vi "Compare Ports.vi"(9 "refresh listbox":T8[](array[typedef]), 10 "new port":T1, 11 "old port":T1) -> (1 "refresh listbox out":T8[](array[typedef]))   [LabVIEW 2020, in "Ballard ARINC 429 System Explorer.lvlib" / "Implementation.lvlib"]
uses:
  Implementation.lvlib
  Types/Refresh Listbox.ctl
  Types/Refresh Symbols.ctl
  Shared/VS Channels Definition for All Labels on Hardware Channel.ctl
  Shared/VS Channels Definition for Label.ctl
  Shared/VS Channel Definition for Parameter.ctl
  Shared/Direction.ctl
  Shared/Parameter Definition.ctl
  Encoding and Decoding/Encoding.ctl
  Shared/Transfer Type.ctl
  Encoding and Decoding/Encoding and Decoding.lvlib
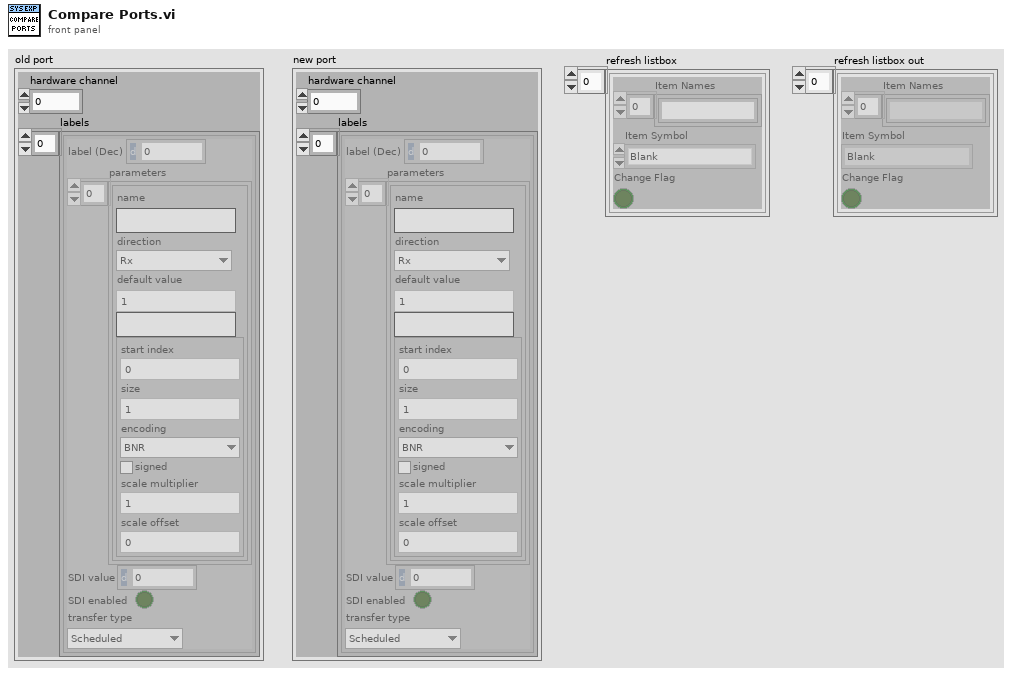
[diagram p1: front panel]
types:
  T1 = typedef "VS Channels Definition for All Labels on Hardware Channel.ctl" = cluster{"hardware channel":i32, "labels":T2[]}
  T2 = typedef "VS Channels Definition for Label.ctl" = cluster{"label (Dec)":u32, "parameters":T3[], "SDI value":u8, "SDI enabled":bool, "transfer type":T7}
  T3 = typedef "VS Channel Definition for Parameter.ctl" = cluster{"name":string, "direction":T4, "default value":dbl, "unit":string, "Parameter":T5}
  T4 = typedef "Direction.ctl" = enum16{"Rx", "Tx"}
  T5 = typedef "Parameter Definition.ctl" = cluster{"start index":i32, "size":i32, "encoding":T6, "signed":bool, "scale multiplier":dbl, "scale offset":dbl}
  T6 = typedef "Encoding and Decoding.lvlib/Encoding.ctl" = enum16{"BNR", "BCD", "Discrete"}
  T7 = typedef "Transfer Type.ctl" = enum16{"Scheduled", "Acyclic", "Block", "Strobe"}
  T8 = typedef "Ballard ARINC 429 System Explorer.lvlib/Implementation.lvlib/Refresh Listbox.ctl" = cluster{"Item Names":string[], "Item Symbol":T9, "Change Flag":bool}
  T9 = typedef "Ballard ARINC 429 System Explorer.lvlib/Implementation.lvlib/Refresh Symbols.ctl" = enum16{"Blank", "Port", "Incoming", "Outgoing", "Label", "Word", "Parameter", "ARINC-429", "Config Files", "Channel Spec", "Item"}
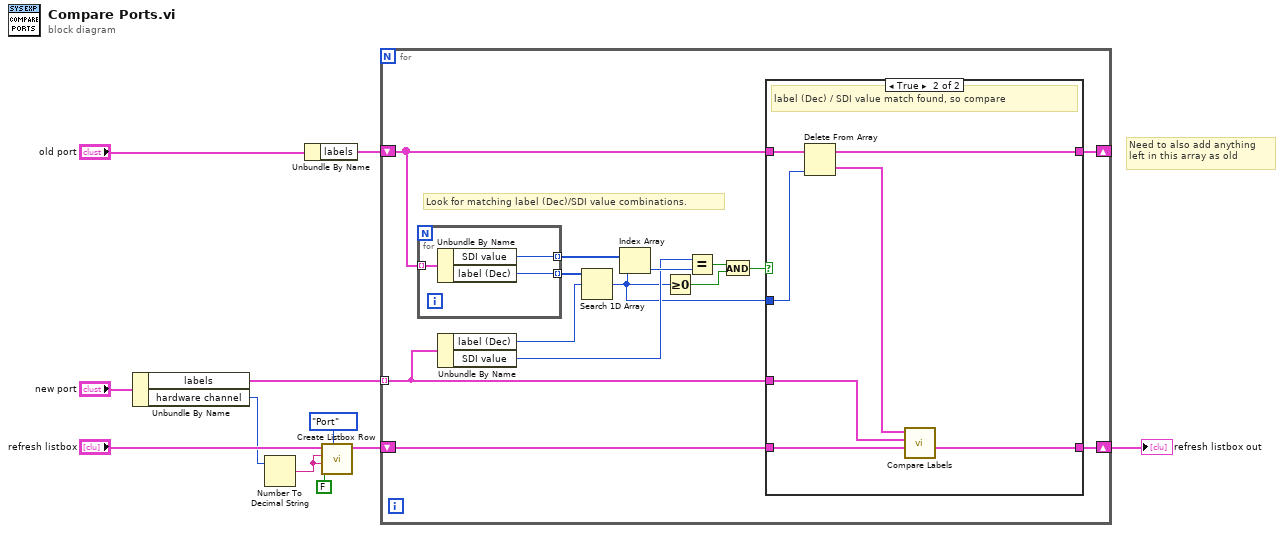
[diagram p0: block diagram]
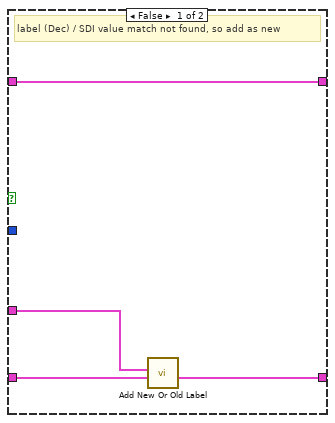
[diagram p2: hidden frame]
diagram:
  # "Need to also add anything left in this array as old"
  n1 = Unbundle By Name("new port") -> ("labels"=w8:T2[], "hardware channel"=w6:i32)
  n2 = Number To Decimal String(number=w6) -> (decimal integer string=w2:string)  [unwired: 1 in]
  n3 = Unbundle By Name("old port") -> ("labels"=w3:T2[])
  n4 = call "Create Listbox Row.vi"("refresh symbol (Blank)"=Refresh_Symbols."Port" ("Refresh Symbol (Blank)"), "change? (T)"=FALSE, "new item"=w2, "old item"=w2, "refresh listbox"="refresh listbox") -> ("refresh listbox out"=w7:T8[])  [unwired: 6 in]
  n5 = for {
    tunnel: w8 -> [w22] mode=indexing
    shift-right: [w24] -> w5
    shift-left: w7 -> [w25]
    shift-right: [w13] -> _
    shift-left: w3 -> [w14]
    # "Look for matching label (Dec)/SDI value combinations."
    n6 = for {
      tunnel: w14 -> [w39] mode=indexing
      tunnel: [w38] -> w23 mode=indexing
      tunnel: [w37] -> w20 mode=indexing
      n7 = Unbundle By Name(w39) -> ("SDI value"=w37:u8, "label (Dec)"=w38:u32)
    }
    n8 = Unbundle By Name(w22) -> ("label (Dec)"=w21:u32, "SDI value"=w18:u8)
    n9 = Search 1D Array(1D array=w23, element=w21) -> (index of element=w12:i32)  [unwired: 1 in]
    n10 = Index Array(array=w20, index=w12) -> (element=w19:u8)
    n11 = Greater Or Equal To 0?(x=w12) -> (x >= 0?=w16:bool)
    n12 = Equal?(x=w18, y=w19) -> (x = y?=w17:bool)
    n13 = And(x=w17, y=w16) -> (x .and. y?=w15:bool)
    n14 = case shown="True" w15 {
      tunnel: w25 -> [w26 w32]
      tunnel: [w27 w33] -> w24
      tunnel: w22 -> [w28 w31]
      tunnel: w14 -> [w29 w36]
      tunnel: [w29 w34] -> w13
      tunnel: w12 -> [_ w35]
      frame False {
        # "label (Dec) / SDI value match not found, so add as new"
        n15 = call "Add New Or Old Label.vi"("refresh listbox"=w26, "label"=w28) -> ("refresh listbox out"=w27:T8[])  [unwired: 9 in]
      }
      frame True {
        # "label (Dec) / SDI value match found, so compare"
        n16 = Delete From Array(array=w36, index=w35) -> (deleted portion=w30:T2, array with subset deleted=w34:T2[])  [unwired: 1 in]
        n17 = call "Compare Labels.vi"("refresh listbox"=w32, "new label"=w31, "old label"=w30) -> ("refresh listbox out"=w33:T8[])  [unwired: 8 in]
      }
    }
  }
  "refresh listbox out" <- w5
